vi "test Add and Get Timing Channels.vi"(8 "error in":errorcluster, 11 "TestCase in":refnum<class "Scripting.lvclass">) -> (0 "error out":errorcluster)   [LabVIEW 2020, in "Scripting.lvclass"]
uses:
  Scripting.lvclass
  C:/Users/nitest/Desktop/Git 2020/niveristand-custom-device-testing-tools/VeriStandScriptingTestCase/VeriStandScriptingTestCase.lvclass
  <vilib>/NI VeriStand/Custom Device API/Custom Device Item Ref.ctl
  niveristand-custom-device-testing-tools/VeriStandScriptingTestCase/VeriStandScriptingTestCase.lvclass/VeriStandScriptingTestCase.ctl
  niveristand-custom-device-testing-tools/VeriStandScriptingTestCase/Read Target.vi
  NationalInstruments.VeriStand.SystemDefinitionAPI
  <vilib>/addons/_JKI Toolkits/VI Tester/TestCase.llb/TestCase.lvclass
  <vilib>/NI VeriStand/Custom Device API/Custom Device API.lvlib
  Scripting/Ballard MIL-STD-1553 Scripting.lvlib
  C:/Program Files (x86)/National Instruments/LabVIEW 2020/vi.lib/addons/_JKI Toolkits/VI Tester/TestCase.llb/TestCase.lvclass
panel:
  out "TestCase out":refnum<class "Scripting.lvclass">
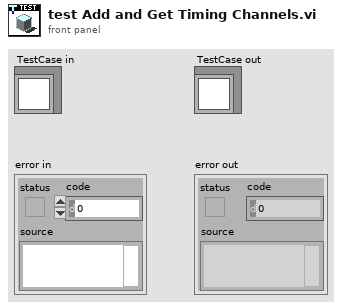
[diagram p1: front panel]
types:
  T1 = typedef "Custom Device API.lvlib/Custom Device Item Ref.ctl" = u64
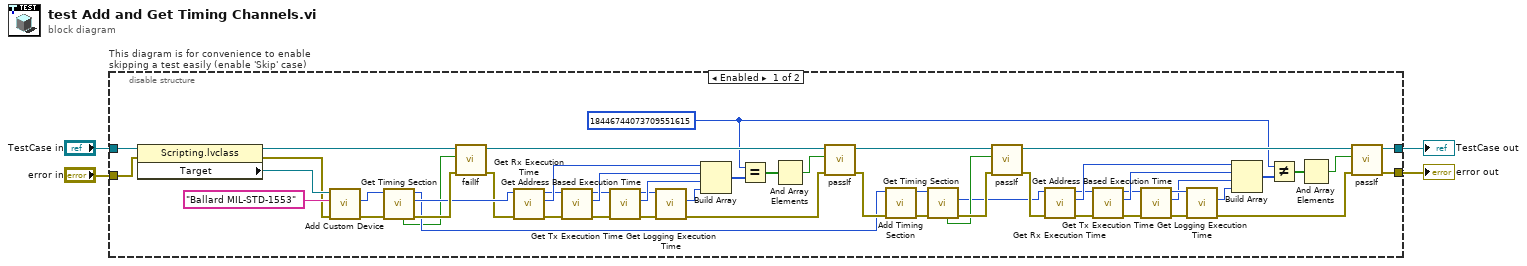
[diagram p0: block diagram]
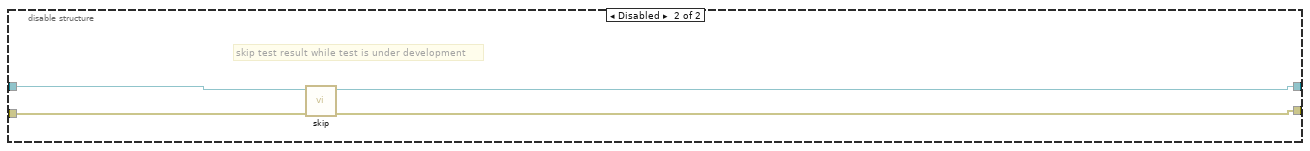
[diagram p2: hidden frame]
diagram:
  n1 = disable-structure "This diagram is for convenience to enable skipping a test easily (enable 'Skip' case)" shown="Enabled" {
    disable-tunnel: "TestCase in" -> [w58 w62]
    disable-tunnel: [w39 w60] -> w1
    disable-tunnel: [w40 w61] -> w3
    disable-tunnel: "error in" -> [w24 w59]
    frame Enabled {
      w28 = T1 18446744073709551615 ("tx acyclic execution time ref")
      n2 = property class="Scripting.lvclass"(reference=w58, error in=w24) -> (reference out=w27:refnum<class "Scripting.lvclass">, error out=w23:errorcluster, "Target"=w26:refnum<k24>)
      n3 = call "Add Custom Device.vi"("error in"=w23, "name"="Ballard MIL-STD-1553", "target in"=w26) -> ("error out"=w22:errorcluster, "Ballard MIL-STD 1553 custom device"=w21:T1)  [unwired: 6 in, 1 out]
      n4 = call "Get Timing Section.vi"("error in"=w22, "custom device in"=w21) -> ("error out"=w57:errorcluster, "timing section out"=w52:T1, "custom device out"=w45:T1, "found"=w38:bool)  [unwired: 6 in]
      n5 = call-dynamic "failIf.vi"("error in (no error)"=w57, "fail"=w38, "TestCase in"=w27) -> ("error out"=w35:errorcluster, "TestCase out"=w51:refnum<class "Scripting.lvclass">)  [unwired: 7 in]
      n6 = call "Get Rx Execution Time.vi"("error in"=w35, "timing section in"=w52) -> ("error out"=w54:errorcluster, "rx execution time"=w49:T1, "timing section out"=w42:T1)  [unwired: 7 in]
      n7 = call "Get Tx Execution Time.vi"("error in"=w54, "timing section in"=w42) -> ("error out"=w53:errorcluster, "tx execution time"=w48:T1, "timing section out"=w41:T1)  [unwired: 7 in]
      n8 = call "Get Address Based Execution Time.vi"("error in"=w53, "timing section in"=w41) -> ("error out"=w50:errorcluster, "address based execution time"=w47:T1, "timing section out"=w9:T1)  [unwired: 7 in]
      n9 = call "Get Logging Execution Time.vi"("error in"=w50, "timing section in"=w9) -> ("error out"=w20:errorcluster, "logging execution time"=w19:T1)  [unwired: 7 in, 1 out]
      n10 = Build Array(w49, w48, w47, w19) -> (w34:T1[])
      n11 = Equal?(x=w28, y=w34) -> (x = y?=w33:bool[])
      n12 = And Array Elements(Boolean array=w33) -> (logical AND=w32:bool)
      n13 = call-dynamic "passIf.vi"("error in (no error)"=w20, "pass"=w32, "TestCase in"=w51) -> ("error out"=w46:errorcluster, "TestCase out"=w44:refnum<class "Scripting.lvclass">)  [unwired: 7 in]
      n14 = call "Add Timing Section.vi"("error in"=w46, "custom device in"=w45) -> ("error out"=w56:errorcluster, "custom device out"=w55:T1)  [unwired: 7 in, 1 out]
      n15 = call "Get Timing Section.vi"("error in"=w56, "custom device in"=w55) -> ("error out"=w43:errorcluster, "timing section out"=w14:T1, "found"=w37:bool)  [unwired: 6 in, 1 out]
      n16 = call-dynamic "passIf.vi"("error in (no error)"=w43, "pass"=w37, "TestCase in"=w44) -> ("error out"=w18:errorcluster, "TestCase out"=w36:refnum<class "Scripting.lvclass">)  [unwired: 7 in]
      n17 = call "Get Rx Execution Time.vi"("error in"=w18, "timing section in"=w14) -> ("error out"=w17:errorcluster, "rx execution time"=w13:T1, "timing section out"=w8:T1)  [unwired: 7 in]
      n18 = call "Get Tx Execution Time.vi"("error in"=w17, "timing section in"=w8) -> ("error out"=w16:errorcluster, "tx execution time"=w12:T1, "timing section out"=w7:T1)  [unwired: 7 in]
      n19 = call "Get Address Based Execution Time.vi"("error in"=w16, "timing section in"=w7) -> ("error out"=w15:errorcluster, "address based execution time"=w5:T1, "timing section out"=w6:T1)  [unwired: 7 in]
      n20 = call "Get Logging Execution Time.vi"("error in"=w15, "timing section in"=w6) -> ("error out"=w10:errorcluster, "logging execution time"=w11:T1)  [unwired: 7 in, 1 out]
      n21 = Build Array(w13, w12, w5, w11) -> (w29:T1[])
      n22 = Not Equal?(x=w28, y=w29) -> (x != y?=w31:bool[])
      n23 = And Array Elements(Boolean array=w31) -> (logical AND=w30:bool)
      n24 = call-dynamic "passIf.vi"("error in (no error)"=w10, "pass"=w30, "TestCase in"=w36) -> ("error out"=w40:errorcluster, "TestCase out"=w39:refnum<class "Scripting.lvclass">)  [unwired: 7 in]
    }
    frame Disabled {
      # "skip test result while test is under development"
      n25 = call <vilib>:"skip.vi"("error in (no error)"=w59, "TestCase in"=w62) -> ("error out"=w61:errorcluster, "TestCase out"=w60:refnum<class "Scripting.lvclass">)  [unwired: 8 in]
    }
  }
  "error out" <- w3
  "TestCase out" <- w1
